vi "Main.vi"() -> ()   [LabVIEW 2020]
doc: "This software acquires data from a simulated source, displays it and performs analysis of the data."
uses:
  Controls/File Type.ctl
  Controls/State.ctl
  Controls/Data.ctl
  Controls/Configuration Settings.ctl
panel:
  in  "File Type":T1
  in  "Open File Location":bool
  in  "Open":bool
  in  "Save":bool
  out "Current State":string
  out "Data":dbl[](graph)
  in  "Reset Settings":bool
  in  "Clear Graph":bool
  in  "Analyze Data":bool
  in  "Acquire Data":bool
  in  "Configure Data":bool
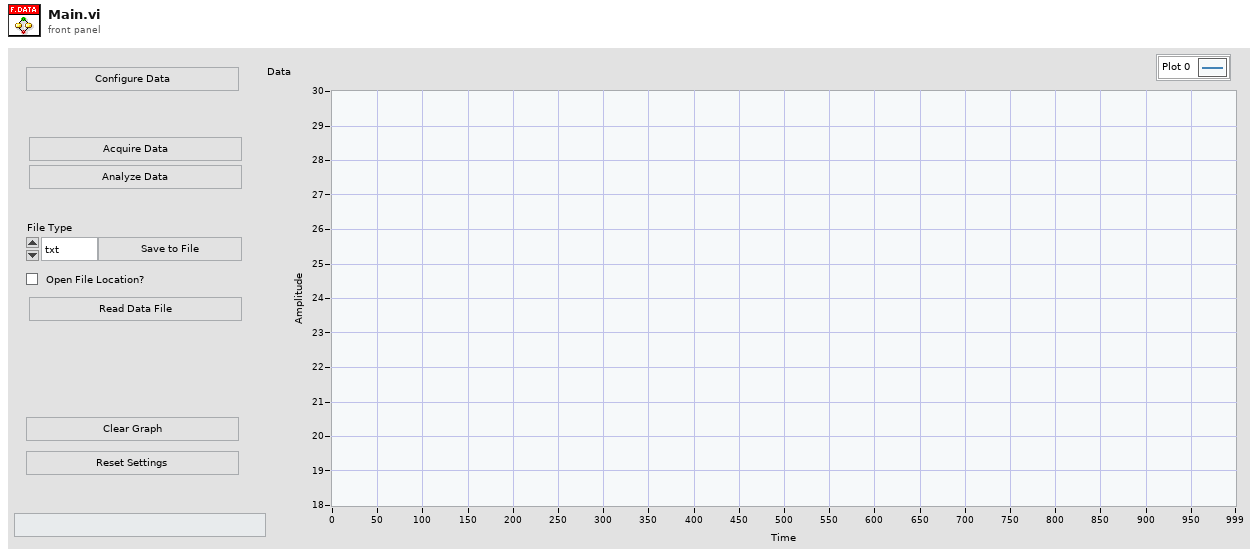
[diagram p1: front panel]
types:
  T1 = typedef "File Type.ctl" = enum16{"txt", "csv", "tdms"}
  T2 = typedef "Data.ctl" = cluster{"Configuration Settings":T3, "Data":dbl[]}
  T3 = typedef "Configuration Settings.ctl" = cluster{"Offset":dbl, "Signal Type":enum16{"Sine Wave", "Triangle Wave", "Square Wave", "Sawtooth Wave"}, "Frequency":dbl, "Amplitude":dbl, "Phase":dbl, "Noise Amplitude":dbl}
  T4 = typedef "State.ctl" = enum16{"Initialize", "Wait for Event", "Configure", "Acquire Data", "Update User Interface", "Reset Data", "Open Data File", "Save Data File", "Clear Data", "Analyse Data", "Stop", "Error"}
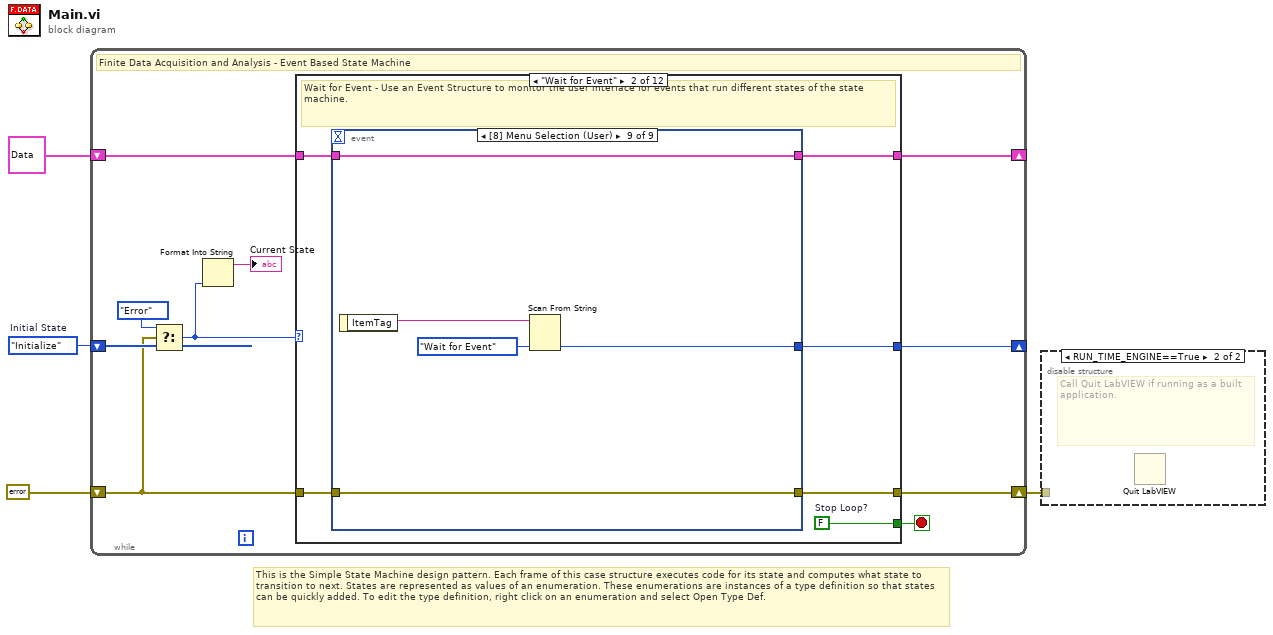
[diagram p0: block diagram]
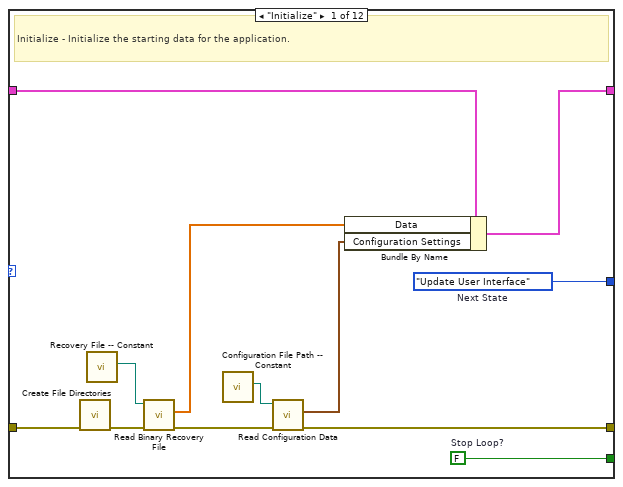
[diagram p2: hidden frame]
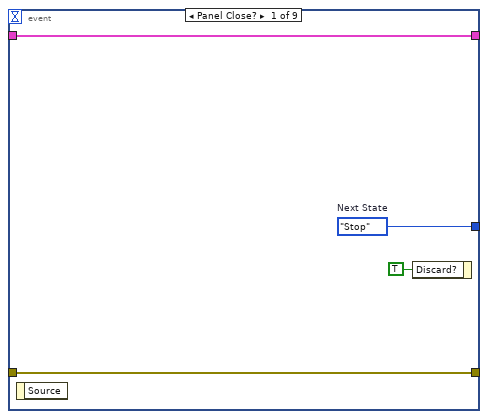
[diagram p3: hidden frame]
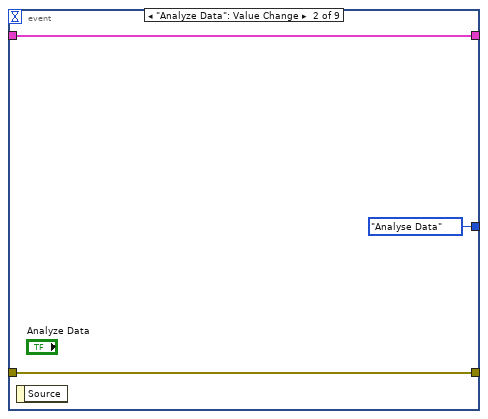
[diagram p4: hidden frame]
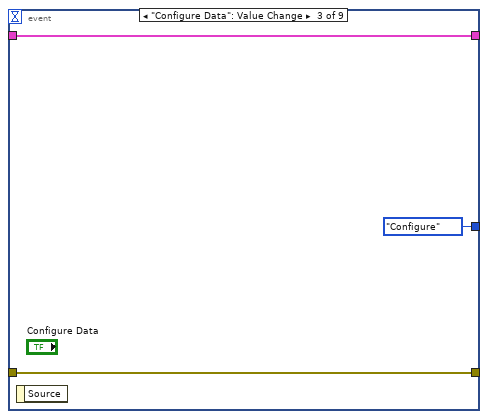
[diagram p5: hidden frame]
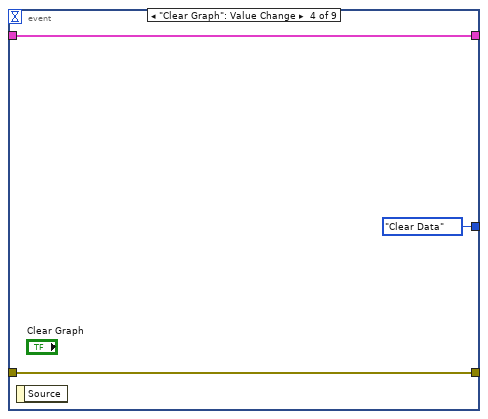
[diagram p6: hidden frame]
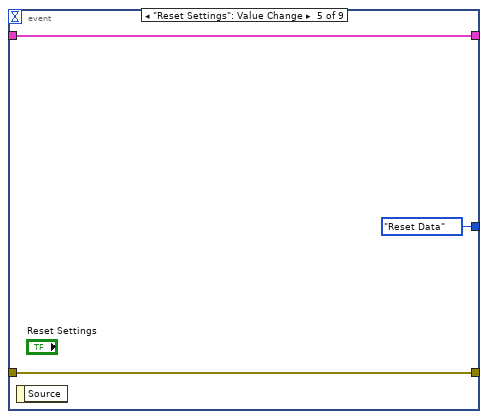
[diagram p7: hidden frame]
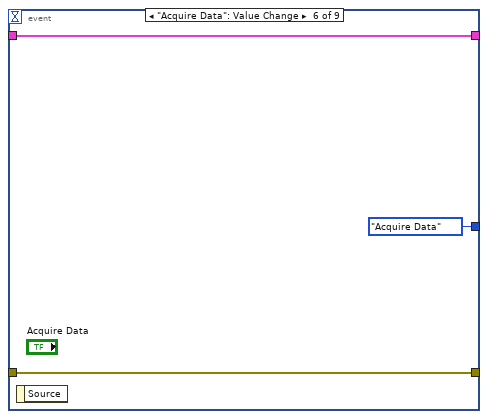
[diagram p8: hidden frame]
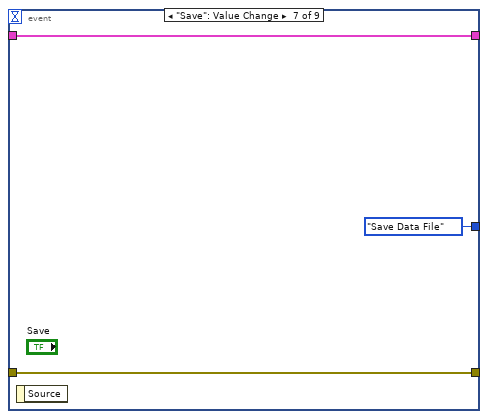
[diagram p9: hidden frame]
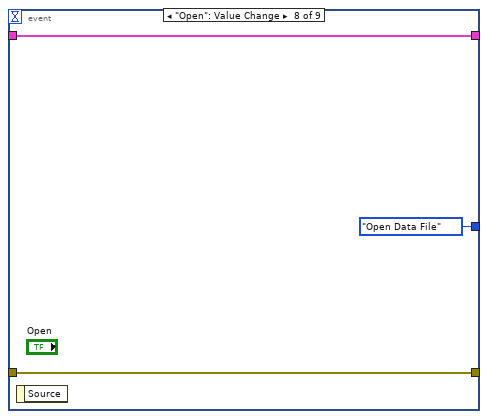
[diagram p10: hidden frame]
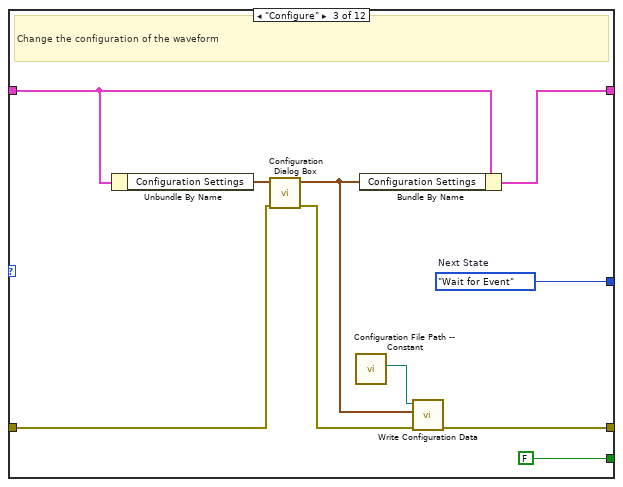
[diagram p11: hidden frame]
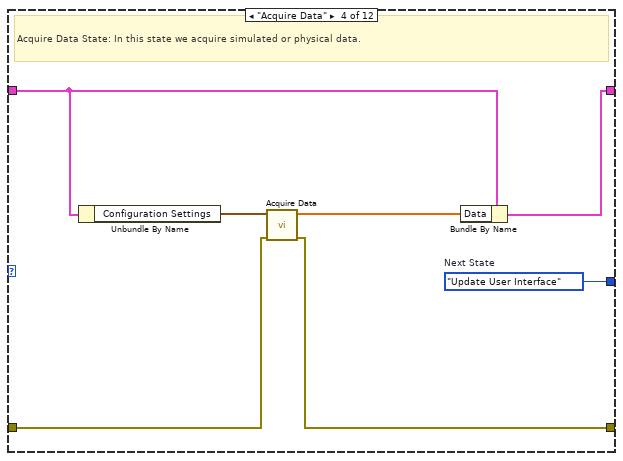
[diagram p12: hidden frame]
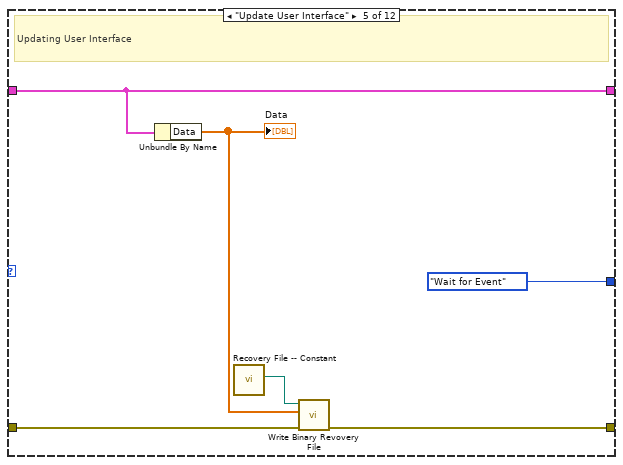
[diagram p13: hidden frame]
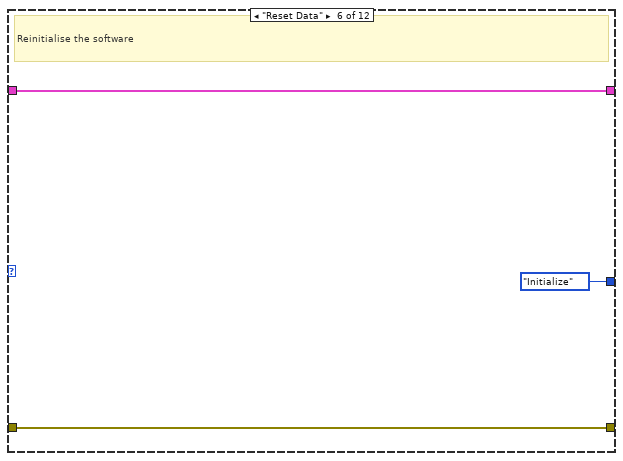
[diagram p14: hidden frame]
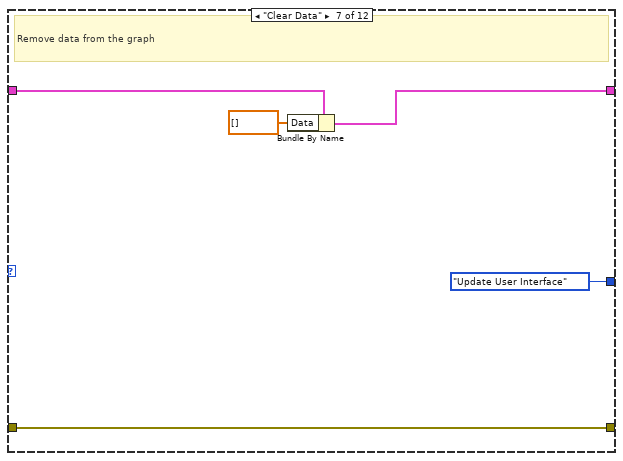
[diagram p15: hidden frame]
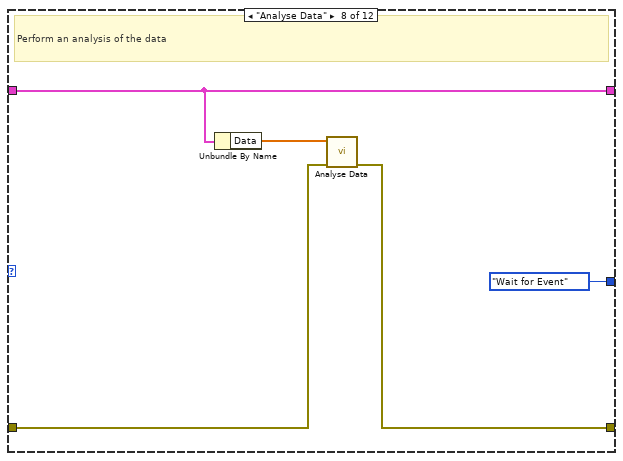
[diagram p16: hidden frame]
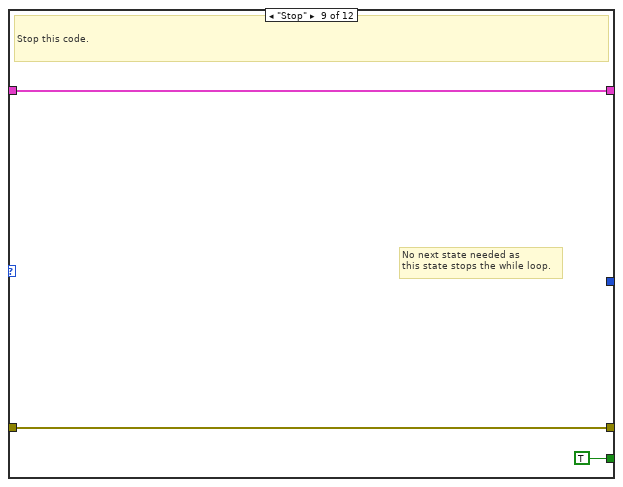
[diagram p17: hidden frame]
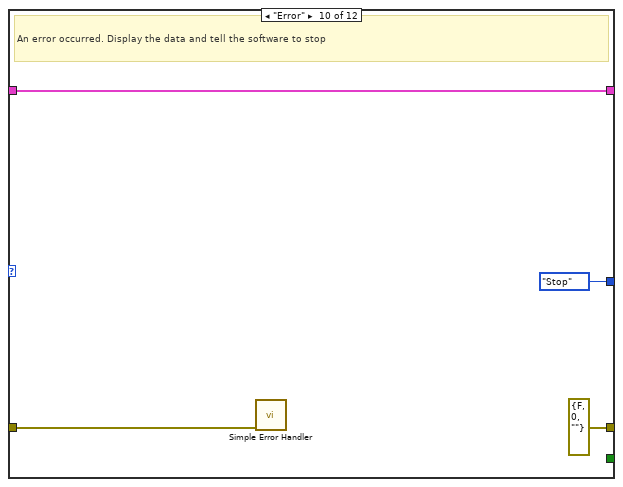
[diagram p18: hidden frame]
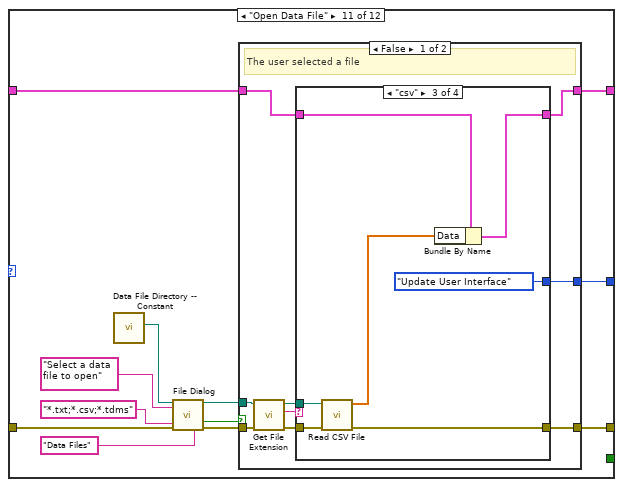
[diagram p19: hidden frame]
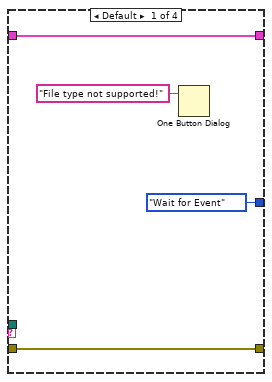
[diagram p20: hidden frame]
diagram:
  w4 = State."Initialize"  # Initial State
  # "This is the Simple State Machine design pattern. Each frame of this case structure executes code for its state and computes what state to transition to next. States are represented as values of an enumeration. These enumerations are instances of a type definition so that states can be quickly added. To edit the type definition, right click on an enumeration and select Open Type Def."
  n1 = while {
    shift-right: [w14] -> _
    shift-left: w4 -> [w9]
    shift-right: [w12] -> _
    shift-left: T2 {"Configuration Settings"={"Offset"=0.0, "Signal Type"=enum."Sine Wave", "Frequency"=10.0, "Amplitude"=1.0, "Phase"=0.0, "Noise Amplitude"=1.0}, "Data"=[]} ("Data") -> [w13]
    shift-right: [w11] -> w1
    shift-left: errorcluster {"status"=FALSE, "code"=0, "source"=""} ("error constant") -> [w10]
    stop <- w5 stop-if-true
    # "Finite Data Acquisition and Analysis - Event Based State Machine"
    n2 = Select(t=State."Error", s=w10, f=w9) -> (s? t:f=w7:T4)
    n3 = Format Into String(w7) -> (resulting string=→"Current State":string)  [unwired: 3 in, 1 out]
    n4 = case shown="\"Wait for Event\"" w7 {
      tunnel: [w26 w32 w72 w79 State."Wait for Event" ("(Value Not Used)") State."Initialize" ("(Value Not Used)") State."Update User Interface" ("(Value Not Used)") State."Wait for Event" ("(Value Not Used)") _ State."Stop" ("(Value Not Used)") w111 State."Wait for Event" ("(Value Not Used)")] -> w14
      tunnel: [w25 w31 FALSE ("Stop Loop?") _ _ _ _ _ TRUE ("Stop Loop?") _ _ _] -> w5
      tunnel: w13 -> [w24 w30 w68 w75 w84 w88 w93 w95 w101 w105 w110 w161]
      tunnel: [w23 w29 w67 w73 w84 w88 w90 w95 w101 w105 w109 w161] -> w12
      tunnel: w10 -> [w19 w28 w70 w78 w82 w87 w92 w97 w100 w103 w117 w157]
      tunnel: [w22 w27 w64 w77 w81 w87 w92 w96 w100 errorcluster {"status"=FALSE, "code"=0, "source"=""} ("error constant") w112 w156] -> w11
      frame "Initialize" {
        w25 = FALSE  # Stop Loop?
        w26 = State."Update User Interface"  # Next State
        # "Initialize - Initialize the starting data for the application."
        n5 = call "Create File Directories.vi"("error in (no error)"=w19) -> ("error out"=w16:errorcluster)  [unwired: 10 in]
        n6 = call "Recovery File -- Constant.vi"() -> ("Recovery File Path"=w15:path)  [unwired: 11 in]
        n7 = call "Read Binary Recovery File.vi"("error in (no error)"=w16, "Path"=w15) -> ("error out"=w17:errorcluster, "Data Out"=w18:dbl[])  [unwired: 8 in]
        n8 = call "Configuration File Path -- Constant.vi"() -> ("Configuration File Path"=w20:path)  [unwired: 11 in]
        n9 = call "Read Configuration Data.vi"("error in (no error)"=w17, "Path"=w20) -> ("error out"=w22:errorcluster, "Configuration Settings"=w21:T3)  [unwired: 8 in]
        n10 = Bundle By Name(cluster=w24, "Data"=w18, "Configuration Settings"=w21) -> (w23:T2)
      }
      frame "Wait for Event" {
        w31 = FALSE  # Stop Loop?
        # "Wait for Event - Use an Event Structure to monitor the user interface for events that run different states of the state machine."
        n11 = event shown="[8] Menu Selection (User)" {
          selector: _ -> [_ _ _ _ _ _ _ _ _]
          dyn-events: _ -> [_ _ _ _ _ _ _ _ _]
          timeout: _ -> [_ _ _ _ _ _ _ _ _]
          tunnel: [w36 State."Analyse Data" ("Next State") State."Configure" ("Next State") State."Clear Data" ("Next State") State."Reset Data" ("Next State") State."Acquire Data" ("Next State") State."Save Data File" ("Next State") State."Open Data File" ("Next State") w58] -> w32
          tunnel: w30 -> [w35 w39 w42 w45 w48 w51 w54 w57 w62]
          tunnel: [w35 w39 w42 w45 w48 w51 w54 w57 w62] -> w29
          tunnel: w28 -> [w34 w38 w41 w44 w47 w50 w53 w56 w61]
          tunnel: [w34 w38 w41 w44 w47 w50 w53 w56 w61] -> w27
          event Panel Close? {
            w36 = State."Stop"  # Next State
            n12 = event-data() -> ()  [unwired: 1 in, 1 out]
            n13 = event-data("Discard?"=TRUE) -> ()  [unwired: 1 in, 1 out]
          }
          event "Analyze Data": Value Change {
            n14 = event-data() -> ()  [unwired: 1 in, 1 out]
          }
          event "Configure Data": Value Change {
            n15 = event-data() -> ()  [unwired: 1 in, 1 out]
          }
          event "Clear Graph": Value Change {
            n16 = event-data() -> ()  [unwired: 1 in, 1 out]
          }
          event "Reset Settings": Value Change {
            n17 = event-data() -> ()  [unwired: 1 in, 1 out]
          }
          event "Acquire Data": Value Change {
            n18 = event-data() -> ()  [unwired: 1 in, 1 out]
          }
          event "Save": Value Change {
            n19 = event-data() -> ()  [unwired: 1 in, 1 out]
          }
          event "Open": Value Change {
            n20 = event-data() -> ()  [unwired: 1 in, 1 out]
          }
          event Menu Selection (User) {
            n21 = event-data() -> ("ItemTag"=w60:string)  [unwired: 1 in]
            n22 = Scan From String(input string=w60, default 1=State."Wait for Event" ("Next State")) -> (output 1=w58:T4)  [unwired: 3 in, 3 out]
          }
        }
      }
      frame "Configure" {
        w72 = State."Wait for Event"  # Next State
        # "Change the configuration of the waveform"
        n23 = Unbundle By Name(w68) -> ("Configuration Settings"=w69:T3)
        n24 = call "Configuration Dialog Box.vi"("error in (no error)"=w70, "Configuration Settings In"=w69) -> ("error out"=w65:errorcluster, "Configuration Settings Out"=w66:T3)  [unwired: 8 in]
        n25 = call "Configuration File Path -- Constant.vi"() -> ("Configuration File Path"=w63:path)  [unwired: 11 in]
        n26 = Bundle By Name(cluster=w68, "Configuration Settings"=w66) -> (w67:T2)
        n27 = call "Write Configuration Data.vi"("error in (no error)"=w65, "Configuration Settings"=w66, "Path"=w63) -> ("error out"=w64:errorcluster)  [unwired: 8 in]
      }
      frame "Acquire Data" {
        w79 = State."Update User Interface"  # Next State
        # "Acquire Data State: In this state we acquire simulated or physical data."
        n28 = Unbundle By Name(w75) -> ("Configuration Settings"=w76:T3)
        n29 = call "Acquire Data.vi"("error in (no error)"=w78, "Configuration Settings"=w76) -> ("error out"=w77:errorcluster, "Data Out"=w74:dbl[])  [unwired: 8 in]
        n30 = Bundle By Name(cluster=w75, "Data"=w74) -> (w73:T2)
      }
      frame "Update User Interface" {
        # "Updating User Interface"
        n31 = Unbundle By Name(w84) -> ("Data"=w83:dbl[])
        "Data" <- w83
        n32 = call "Recovery File -- Constant.vi"() -> ("Recovery File Path"=w80:path)  [unwired: 11 in]
        n33 = call "Write Binary Revovery File.vi"("error in (no error)"=w82, "Data In"=w83, "Path"=w80) -> ("error out"=w81:errorcluster)  [unwired: 8 in]
      }
      frame "Reset Data" {
        # "Reinitialise the software"
      }
      frame "Clear Data" {
        # "Remove data from the graph"
        n34 = Bundle By Name(cluster=w93, "Data"=dbl[] []) -> (w90:T2)
      }
      frame "Analyse Data" {
        # "Perform an analysis of the data"
        n35 = Unbundle By Name(w95) -> ("Data"=w94:dbl[])
        n36 = call "Analyse Data.vi"("error in (no error)"=w97, "Data In"=w94) -> ("error out"=w96:errorcluster)  [unwired: 9 in]
      }
      frame "Stop" {
        # "No next state needed as \nthis state stops the while loop."
        # "Stop this code."
      }
      frame "Error" {
        # "An error occurred. Display the data and tell the software to stop"
        n37 = call <vilib>:"Simple Error Handler.vi"("error in (no error)"=w103) -> ()  [unwired: 4 in, 5 out]
      }
      frame "Open Data File" {
        n38 = call "Data File Directory -- Constant.vi"() -> ("Data File Directory"=w106:path)  [unwired: 11 in]
        n39 = call "File Dialog"("start path"=w106, "prompt"="Select a data file to open", "error in"=w117, "pattern (all files)"="*.txt;*.csv;*.tdms", "pattern label"="Data Files") -> ("selected path"=w108:path, "cancelled"=w113:bool, "error out"=w107:errorcluster)  [unwired: 7 in, 1 out]
        n40 = case shown="False" w113 {
          tunnel: [w123 w154] -> w112
          tunnel: [w124 State."Wait for Event" ("t")] -> w111
          tunnel: w110 -> [w126 w152]
          tunnel: [w125 w152] -> w109
          tunnel: w108 -> [w121 _]
          tunnel: w107 -> [w120 _]
          frame False {
            # "The user selected a file"
            n41 = call <vilib>:"Get File Extension.vi"("error in (no error)"=w120, "file"=w121) -> ("error out"=w122:errorcluster, "lowercase file extension"=w119:string, "dup file"=w118:path)  [unwired: 5 in, 2 out]
            n42 = case shown="\"csv\"" w119 {
              tunnel: w126 -> [w130 w137 w144 w151]
              tunnel: [w130 w136 w143 w150] -> w125
              tunnel: [State."Wait for Event" ("t") State."Update User Interface" ("t") State."Update User Interface" ("t") State."Update User Interface" ("t")] -> w124
              tunnel: [w127 w132 w138 w146] -> w123
              tunnel: w122 -> [w127 w133 w140 w147]
              tunnel: w118 -> [_ w134 w141 w148]
              frame Default {
                n43 = One Button Dialog(message="File type not supported!") -> ()  [unwired: 1 in, 1 out]
              }
              frame "tdms" {
                n44 = call "Read TDMS File.vi"("error in (no error)"=w133, "Path"=w134) -> ("error out"=w132:errorcluster, "Data"=w131:dbl[])  [unwired: 8 in]
                n45 = Bundle By Name(cluster=w137, "Data"=w131) -> (w136:T2)
              }
              frame "csv" {
                n46 = call "Read CSV File.vi"("error in (no error)"=w140, "Path"=w141) -> ("error out"=w138:errorcluster, "Data"=w139:dbl[])  [unwired: 8 in]
                n47 = Bundle By Name(cluster=w144, "Data"=w139) -> (w143:T2)
              }
              frame "txt" {
                n48 = call "Read Text File.vi"("error in (no error)"=w147, "Path"=w148) -> ("error out"=w146:errorcluster, "Data"=w145:dbl[])  [unwired: 8 in]
                n49 = Bundle By Name(cluster=w151, "Data"=w145) -> (w150:T2)
              }
            }
          }
          frame True {
            # "The user cancelled the file dialog"
            n50 = call <vilib>:"Clear Errors.vi"("specific error code to clear (0: all)"=43) -> ("error out"=w154:errorcluster)  [unwired: 5 in, 1 out]
          }
        }
      }
      frame "Save Data File" {
        n51 = Unbundle By Name(w161) -> ("Data"=w159:dbl[])
        n52 = call "Save Data File.vi"("error in (no error)"=w157, "Open File Location"="Open File Location", "Data"=w159, "File Type"="File Type") -> ("error out"=w156:errorcluster)  [unwired: 7 in]
      }
    }
  }
  n53 = disable-structure shown="RUN_TIME_ENGINE==True" {
    disable-tunnel: w1 -> [_ _]
    frame condition #0 (active) {
    }
    frame condition #1 {
      # "Call Quit LabVIEW if running as a built application."
      n54 = Quit LabVIEW() -> ()  [unwired: 1 in]
    }
  }
